vi "Value Change.vi"(10 "Tree Tag":string, 11 "UI Data In":refnum<class "Settings UI.lvclass">) -> (3 "UI Data Out":refnum<class "Settings UI.lvclass">)   [LabVIEW 2020, in "Output Sequencer.lvlib" / "Settings UI.lvclass"]
uses:
  Settings UI.lvclass
  Types/Data Type.ctl
  Settings UI.lvclass/Settings UI.ctl
  Types/Data Type Enum.ctl
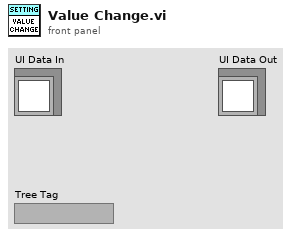
[diagram p1: front panel]
types:
  T1 = typedef "Output Sequencer.lvlib/Settings UI.lvclass/Data Type.ctl" = i16
  T2 = typedef "Output Sequencer.lvlib/Settings UI.lvclass/Tree Item Settings.ctl" = cluster{"Tree Label":string, "Indent Level":i32, "Data Type":T1, "Numeric Range":cluster{"Min":dbl, "Max":dbl, "Inc":dbl}, "Allowed Values":string[], "Default Value":string, "Description":string}
  T3 = typedef "Output Sequencer.lvlib/Settings UI.lvclass/Data Type Enum.ctl" = enum16{"Numeric", "String", "Boolean", "Enum"}
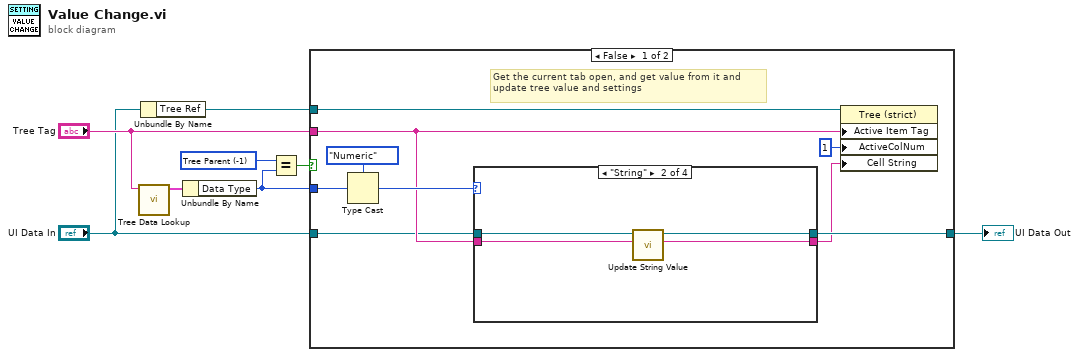
[diagram p0: block diagram]
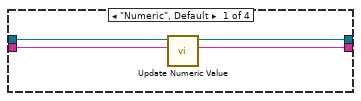
[diagram p2: hidden frame]
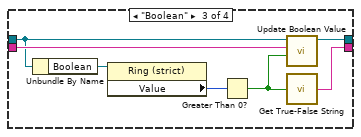
[diagram p3: hidden frame]
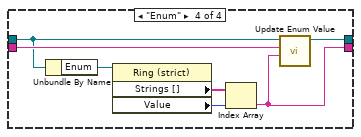
[diagram p4: hidden frame]
diagram:
  w2 = T1 -1 items=["Tree Parent"=-1, "Numeric"=0, "String"=1, "Boolean"=2, "Enum"=3] ("Data Type")
  n1 = call "Tree Data Lookup.vi"("Tag in"="Tree Tag") -> ("Tree Data"=w3:T2)  [unwired: 5 in, 5 out]
  n2 = Unbundle By Name("UI Data In") -> ("Tree Ref"=w8:refnum<vi>)
  n3 = Unbundle By Name(w3) -> ("Data Type"=w5:T1)
  n4 = Equal?(x=w2, y=w5) -> (x = y?=w6:bool)
  n5 = case shown="False" w6 {
    tunnel: w8 -> [w14 _]
    tunnel: "Tree Tag" -> [w13 _]
    tunnel: w5 -> [w17 _]
    tunnel: "UI Data In" -> [w12 w40]
    tunnel: [w11 w40] -> w4
    frame False {
      # "Get the current tab open, and get value from it and update tree value and settings"
      n6 = Type Cast(type=Data_Type_Enum."Numeric" ("Data Type"), x=w17) -> (*(type *) &x=w15:T3)
      n7 = case shown="\"String\"" w15 {
        tunnel: [w19 w22 w27 w36] -> w10
        tunnel: w13 -> [w18 w23 w29 w34]
        tunnel: w12 -> [w21 w25 w26 w33]
        tunnel: [w20 w24 w30 w35] -> w11
        frame "Numeric", Default {
          n8 = call "Update Numeric Value.vi"("Tree Tag"=w18, "UI Data In"=w21) -> ("New Tree Value"=w19:string, "UI Data out"=w20:refnum<class "Settings UI.lvclass">)  [unwired: 8 in]
        }
        frame "String" {
          n9 = call "Update String Value.vi"("Tree Tag"=w23, "UI Data In"=w25) -> ("New Tree Value"=w22:string, "UI Data Out"=w24:refnum<class "Settings UI.lvclass">)  [unwired: 8 in]
        }
        frame "Boolean" {
          n10 = Unbundle By Name(w26) -> ("Boolean"=w32:refnum<vi>)
          n11 = property class="Ring (strict)"(reference=w32) -> ("Value"=w31:u16)  [unwired: 1 in, 2 out]
          n12 = Greater Than 0?(x=w31) -> (x > 0?=w28:bool)
          n13 = call "Update Boolean Value.vi"("Value"=w28, "Tree Tag"=w29, "UI Data in"=w26) -> ("UI Data out"=w30:refnum<class "Settings UI.lvclass">)  [unwired: 8 in]
          n14 = call "Get True-False String.vi"("Input"=w28) -> ("True/False String"=w27:string)
        }
        frame "Enum" {
          n15 = Unbundle By Name(w33) -> ("Enum"=w37:refnum<vi>)
          n16 = property class="Ring (strict)"(reference=w37) -> ("Strings []"=w39:string[], "Value"=w38:u16)  [unwired: 1 in, 2 out]
          n17 = Index Array(array=w39, index=w38) -> (element=w36:string)
          n18 = call "Update Enum Value.vi"("Value"=w36, "Tree Tag"=w34, "UI Data In"=w33) -> ("UI Data Out"=w35:refnum<class "Settings UI.lvclass">)  [unwired: 8 in]
        }
      }
      n19 = property class="Tree (strict)"(reference=w14, "Active Item Tag"=w13, "ActiveColNum"=1 ("Active Cell:Active Column Number"), "Cell String"=w10) -> ()  [unwired: 1 in, 2 out]
    }
    frame True {
    }
  }
  "UI Data Out" <- w4
